vi "ShooterB Test2.vi"(2 "GetMotorOut":dbl, 3 "Encoder":dbl, 4 "Shooter":dbl) -> (0 "CurrentSpeed":dbl, 1 "ToMotor":dbl)   [LabVIEW 2011]
uses:
  Robot Global Data.vi
panel:
  out "Waveform Chart":dbl(graph)
  out "TimeForRange":dbl
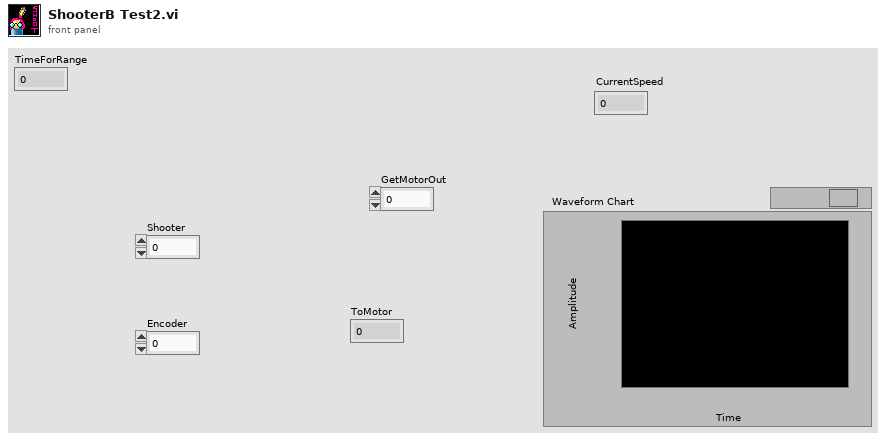
[diagram p1: front panel]
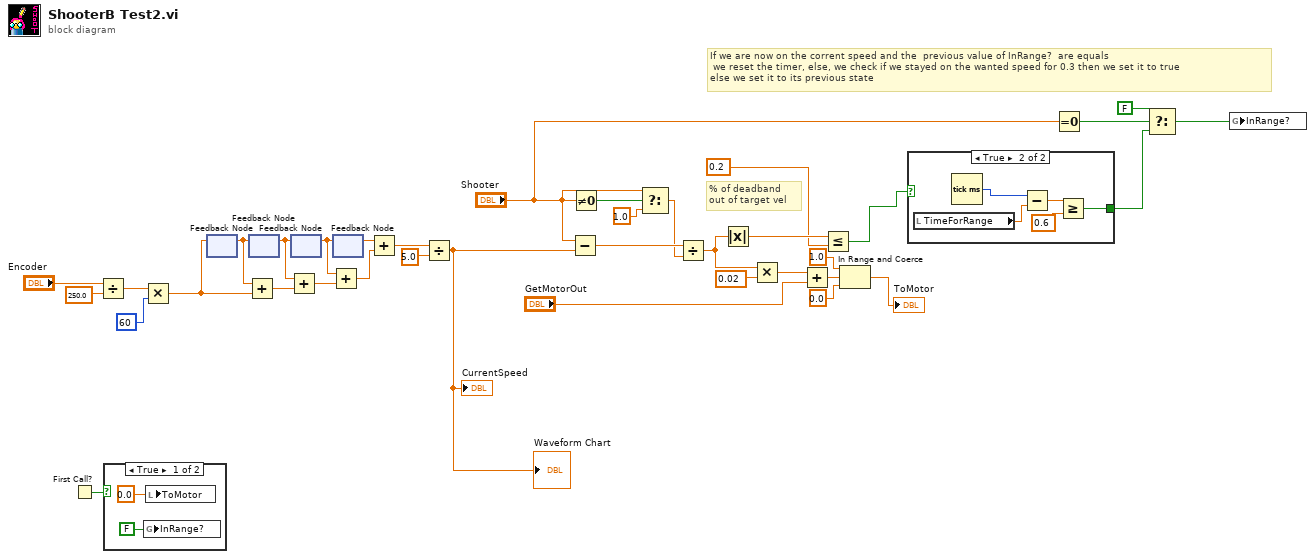
[diagram p0: block diagram]
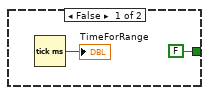
[diagram p2: hidden frame]
diagram:
  # "% of deadband\nout of target vel"
  # "If we are now on the corrent speed and the  previous value of InRange?  are equals\n we reset the timer, else, we check if we stayed on the wanted speed for 0.3 then we set it to true\nelse we set it to its previous state"
  n1 = First Call?() -> (First Call?: T/F=w33:bool)
  n2 = Divide(x="Encoder", y=250.0) -> (x/y=w31:dbl)
  n3 = case shown="True" w33 {
    frame True {
      n4 = global write "Robot Global Data.vi" "InRange?"(FALSE ("InRange?")) -> ()
      n5 = local write "ToMotor"(0.0 ("ToMotor")) -> ()
    }
    frame False {
    }
  }
  n6 = Multiply(x=w31, y=60) -> (x*y=w30:dbl)
  n7 = feedback #1() -> (w21:dbl)  [unwired: 1 in]
  n8 = feedback-in #1(w30) -> ()
  n9 = Add(x=w21, y=w30) -> (x+y=w20:dbl)
  n10 = feedback #2() -> (w25:dbl)  [unwired: 1 in]
  n11 = feedback-in #2(w21) -> ()
  n12 = Add(x=w25, y=w20) -> (x+y=w26:dbl)
  n13 = feedback #3() -> (w23:dbl)  [unwired: 1 in]
  n14 = feedback-in #3(w25) -> ()
  n15 = Add(x=w23, y=w26) -> (x+y=w24:dbl)
  n16 = feedback #4() -> (w22:dbl)  [unwired: 1 in]
  n17 = feedback-in #4(w23) -> ()
  n18 = Add(x=w22, y=w24) -> (x+y=w27:dbl)
  n19 = Divide(x=w27, y=5.0) -> (x/y=w1:dbl)
  "CurrentSpeed" <- w1
  "Waveform Chart" <- w1
  n20 = Subtract(x="Shooter", y=w1) -> (x-y=w17:dbl)
  n21 = Not Equal To 0?(x="Shooter") -> (x != 0?=w15:bool)
  n22 = Select(t="Shooter", s=w15, f=1.0) -> (s? t:f=w14:dbl)
  n23 = Divide(x=w17, y=w14) -> (x/y=w12:dbl)
  n24 = Absolute Value(x=w12) -> (abs(x)=w11:dbl)
  n25 = Multiply(x=w12, y=0.02) -> (x*y=w16:dbl)
  n26 = Add(x=w16, y="GetMotorOut") -> (x+y=w18:dbl)
  n27 = Less Or Equal?(x=w11, y=0.2) -> (x <= y?=w32:bool)
  n28 = In Range and Coerce(upper limit=1.0, x=w18, lower limit=0.0) -> (coerced(x)=→"ToMotor":dbl)  [unwired: 1 out]
  n29 = case shown="True" w32 {
    tunnel: [FALSE w41] -> w3
    frame False {
      n30 = Tick Count (ms)() -> (millisecond timer value=→"TimeForRange":u32)
    }
    frame True {
      n31 = local read "TimeForRange"() -> (w44:dbl)
      n32 = Tick Count (ms)() -> (millisecond timer value=w45:u32)
      n33 = Subtract(x=w45, y=w44) -> (x-y=w43:dbl)
      n34 = Greater Or Equal?(x=w43, y=0.6) -> (x >= y?=w41:bool)
    }
  }
  n35 = Equal To 0?(x="Shooter") -> (x = 0?=w6:bool)
  n36 = Select(t=FALSE, s=w6, f=w3) -> (s? t:f=w2:bool)
  n37 = global write "Robot Global Data.vi" "InRange?"(w2) -> ()
